vi "Energy_Estimation.vi"(9 "Energy Total":dbl(knob) scale=0.0..10.0, 11 "Signal Out":dbl(knob) scale=0.0..10.0) -> (1 "Energy Out":dbl)   [LabVIEW 2014]
panel:
  # "Omega Power Usage Estimation"
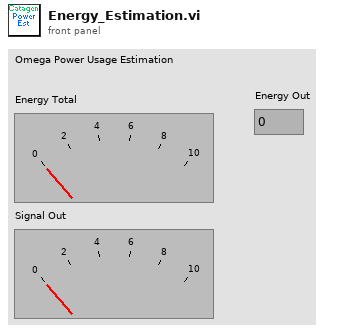
[diagram p1: front panel]
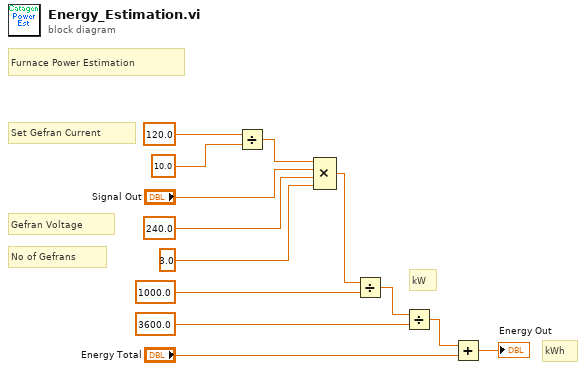
[diagram p0: block diagram]
diagram:
  # "kW"
  # "kWh"
  # "No of Gefrans"
  # "Gefran Voltage"
  # "Set Gefran Current"
  # "Furnace Power Estimation"
  n1 = Divide(x=120.0, y=10.0) -> (x/y=w11:dbl)
  n2 = Compound Arithmetic op=MULTIPLY(w11, "Signal Out", 240.0 ("x"), 3.0 ("x")) -> (w7:dbl)
  n3 = Divide(x=w7, y=1000.0) -> (x/y=w4:dbl)
  n4 = Divide(x=w4, y=3600.0) -> (x/y=w3:dbl)
  n5 = Add(x=w3, y="Energy Total") -> (x+y=→"Energy Out":dbl)
